vi "Add Engine Simulation Toolkit Custom Device.vi"(8 "error in (no error)":errorcluster, 10 "Settings":T1={"Name"="", "Execution priority"=enum."Medium", "Rate decimation"=1, "CPU"=-2} {"Rate decimation" min=1}, 11 "Target in":refnum<k24>) -> (0 "error out":errorcluster, 2 "EST Custom Device":refnum<k24>, 3 "Target out":refnum<k24>)   [LabVIEW 2015, in "Engine Simulation Toolkit Scripting API.lvlib"]
uses:
  Engine Simulation Toolkit Scripting API.lvlib
  NationalInstruments.VeriStand.SystemDefinitionAPI
  Engine Simulation Toolkit Custom Device Settings.ctl
  Shared/Constants and GUIDs.vi
  Shared/Engine Simulation Toolkit Shared.lvlib
  System Explorer/Engine Simulation Toolkit System Explorer.lvlib
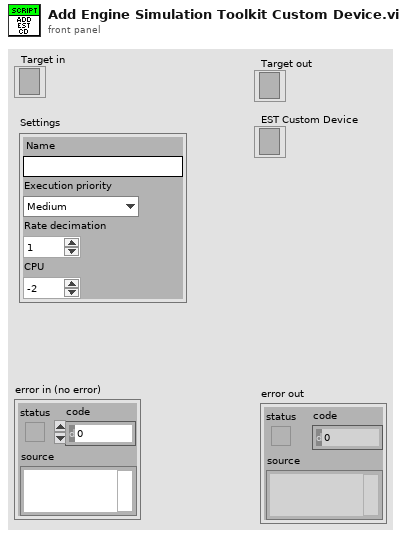
[diagram p1: front panel]
types:
  T1 = typedef "Engine Simulation Toolkit Scripting API.lvlib/Engine Simulation Toolkit Custom Device Settings.ctl" = cluster{"Name":string, "Execution priority":enum16{"Low", "Medium", "High"}, "Rate decimation":i32, "CPU":i32}
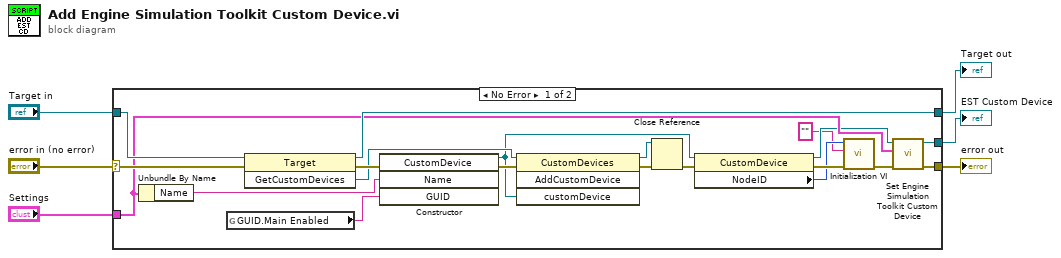
[diagram p0: block diagram]
diagram:
  n1 = case shown="No Error" "error in (no error)" {
    selector: "error in (no error)" -> [w26 w28]
    tunnel: [w16 w28] -> w6
    tunnel: "Target in" -> [w25 w27]
    tunnel: [w20 w27] -> w3
    tunnel: "Settings" -> [w14 _]
    tunnel: [w17 _] -> w1
    frame No Error {
      n2 = Unbundle By Name(w14) -> ("Name"=w15:string)
      n3 = global read "Constants and GUIDs.vi" "GUID.Main Enabled"() -> (w23:string)
      n4 = invoke class="Target" method="GetCustomDevices"(reference=w25, error in=w26) -> (reference out=w20:refnum<k24>, error out=w24:errorcluster, "GetCustomDevices"=w22:refnum<k24>)  [unwired: 1 in]
      n5 = constructor class="CustomDevice"(error in=w24, "Name"=w15, "GUID"=w23) -> (reference out=w13:refnum<k24>, error out=w21:errorcluster)  [unwired: 2 in, 3 out]
      n6 = invoke class="CustomDevices" method="AddCustomDevice"(reference=w22, error in=w21, "customDevice"=w13) -> (reference out=w19:refnum<k24>, error out=w18:errorcluster)  [unwired: 1 in, 2 out]
      n7 = Close Reference(reference=w19, error in (no error)=w18) -> (error out=w11:errorcluster)
      n8 = property class="CustomDevice"(reference=w13, error in=w11) -> (reference out=w12:refnum<k24>, error out=w10:errorcluster, "NodeID"=w8:u64)
      n9 = call "Initialization VI.vi"("error in (no error)"=w10, "Custom XML"="", "Device Item Ref in"=w8) -> ("error out"=w9:errorcluster)  [unwired: 7 in, 1 out]
      n10 = call "Set Engine Simulation Toolkit Custom Device.vi"("error in (no error)"=w9, "Settings"=w14, "EST Custom Device in"=w12) -> ("error out"=w16:errorcluster, "EST Custom Device out"=w17:refnum<k24>)  [unwired: 7 in]
    }
    frame Error {
    }
  }
  "Target out" <- w3
  "error out" <- w6
  "EST Custom Device" <- w1
